vi "RSZVB Set IMOD Two Tone Output.vi"(8 "error in (no error)":errorcluster {"code" format="%.0x"}, 9 "Two Tone Output (1)":i32(ring)=1 items=["Port", "External device"], 10 "Channel (1)":i32=1, 11 "VISA session":refnum<visa-resource-name>) -> (0 "error out":errorcluster {"code" format="%.0x"}, 3 "dup VISA session":refnum<visa-resource-name>)   [LabVIEW 2011]
doc: "Selects the source for the two tone output signal for intermodulation measurements.\n\nRemote-control command(s):\n[SENSe<Ch>:]FREQuency:IMODulation:TTOutput PORT | EDEVice"
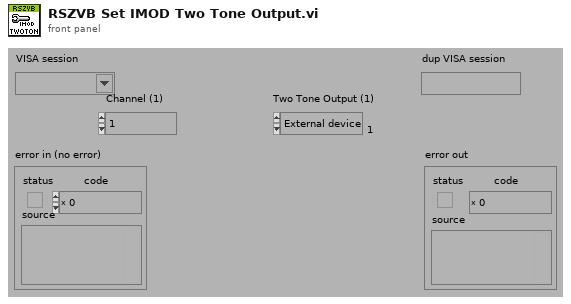
[diagram p1: front panel]
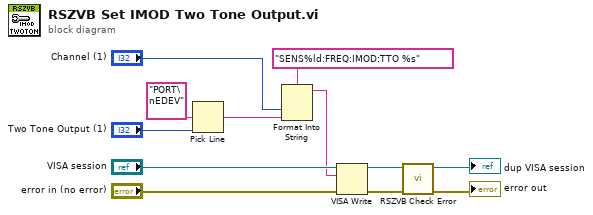
[diagram p0: block diagram]
diagram:
  n1 = Pick Line(multi-line string="PORT\nEDEV", line index="Two Tone Output (1)") -> (output string=w8:string)  [unwired: 1 in]
  n2 = Format Into String(format string="SENS%ld:FREQ:IMOD:TTO %s", "Channel (1)", w8) -> (resulting string=w5:string)  [unwired: 2 in, 1 out]
  n3 = VISA Write(VISA resource name="VISA session", write buffer=w5, error in (no error)="error in (no error)") -> (VISA resource name out=w3:refnum<visa-resource-name>, error out=w4:errorcluster)  [unwired: 1 out]
  n4 = call "RSZVB Check Error.vi"("error in (no error)"=w4, "VISA session"=w3) -> ("error out"=→"error out":errorcluster, "dup VISA session"=→"dup VISA session":refnum<visa-resource-name>)  [unwired: 8 in]
